vi "test_Set-Get Protocol ConvBox.vi"(8 "error in (no error)":errorcluster, 11 "TestCase in":refnum<class "Instrument Addon Scripting API Custom Device Unit Tests.lvclass">) -> (0 "error out":errorcluster, 3 "TestCase out":refnum<class "Instrument Addon Scripting API Custom Device Unit Tests.lvclass">)   [LabVIEW 2018, in "Instrument Addon Scripting API Custom Device Unit Tests.lvclass"]
uses:
  Instrument Addon Scripting API Custom Device Unit Tests.lvclass
  Addon/Support Libraries/Protocols.lvlibp/RS-xxx to GPIB ConvBox/RS-xxx to GPIB ConvBox.lvclass
  C:/Users/nitest/Git/NI VS Instrument Addon Fork/Source/Addon/Support Libraries/Protocols.lvlibp/Protocol Parent/Protocol Parent.lvclass
  Addon/Support Libraries/Protocols.lvlibp/TCP/TCP.lvclass
  Addon/Support Libraries/Protocols.lvlibp/RS-xxx to GPIB ConvBox/Data Access/Write Assert Ren with IFC.vi
  Addon/Support Libraries/Protocols.lvlibp/RS-xxx to GPIB ConvBox/Data Access/Write ConvBox Address.vi
  Addon/Support Libraries/Protocols.lvlibp/RS-xxx to GPIB ConvBox/Data Access/Write GPIB Address.vi
  Addon/Support Libraries/Protocols.lvlibp/RS-xxx to GPIB ConvBox/Data Access/Write IST bit sense.vi
  Addon/Support Libraries/Protocols.lvlibp/RS-xxx to GPIB ConvBox/Data Access/Write Port.vi
  Addon/Support Libraries/Protocols.lvlibp/RS-xxx to GPIB ConvBox/Data Access/Write System controller.vi
  Instrument Addon Scripting API Test Assets/Instrument Addon Scripting API Test Assets.lvclass
  <vilib>/addons/_JKI Toolkits/VI Tester/TestCase.llb/TestCase.lvclass
  APIs/Scripting API/Instrument Addon Scripting API.lvlib
  C:/Program Files (x86)/National Instruments/LabVIEW 2018/vi.lib/addons/_JKI Toolkits/VI Tester/TestCase.llb/TestCase.lvclass
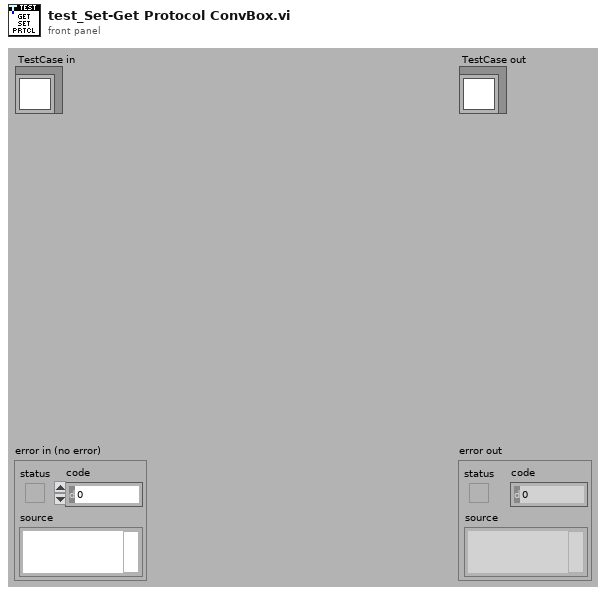
[diagram p1: front panel]
types:
  T1 = typedef "Custom Device API.lvlib/Custom Device Item Ref.ctl" = u64
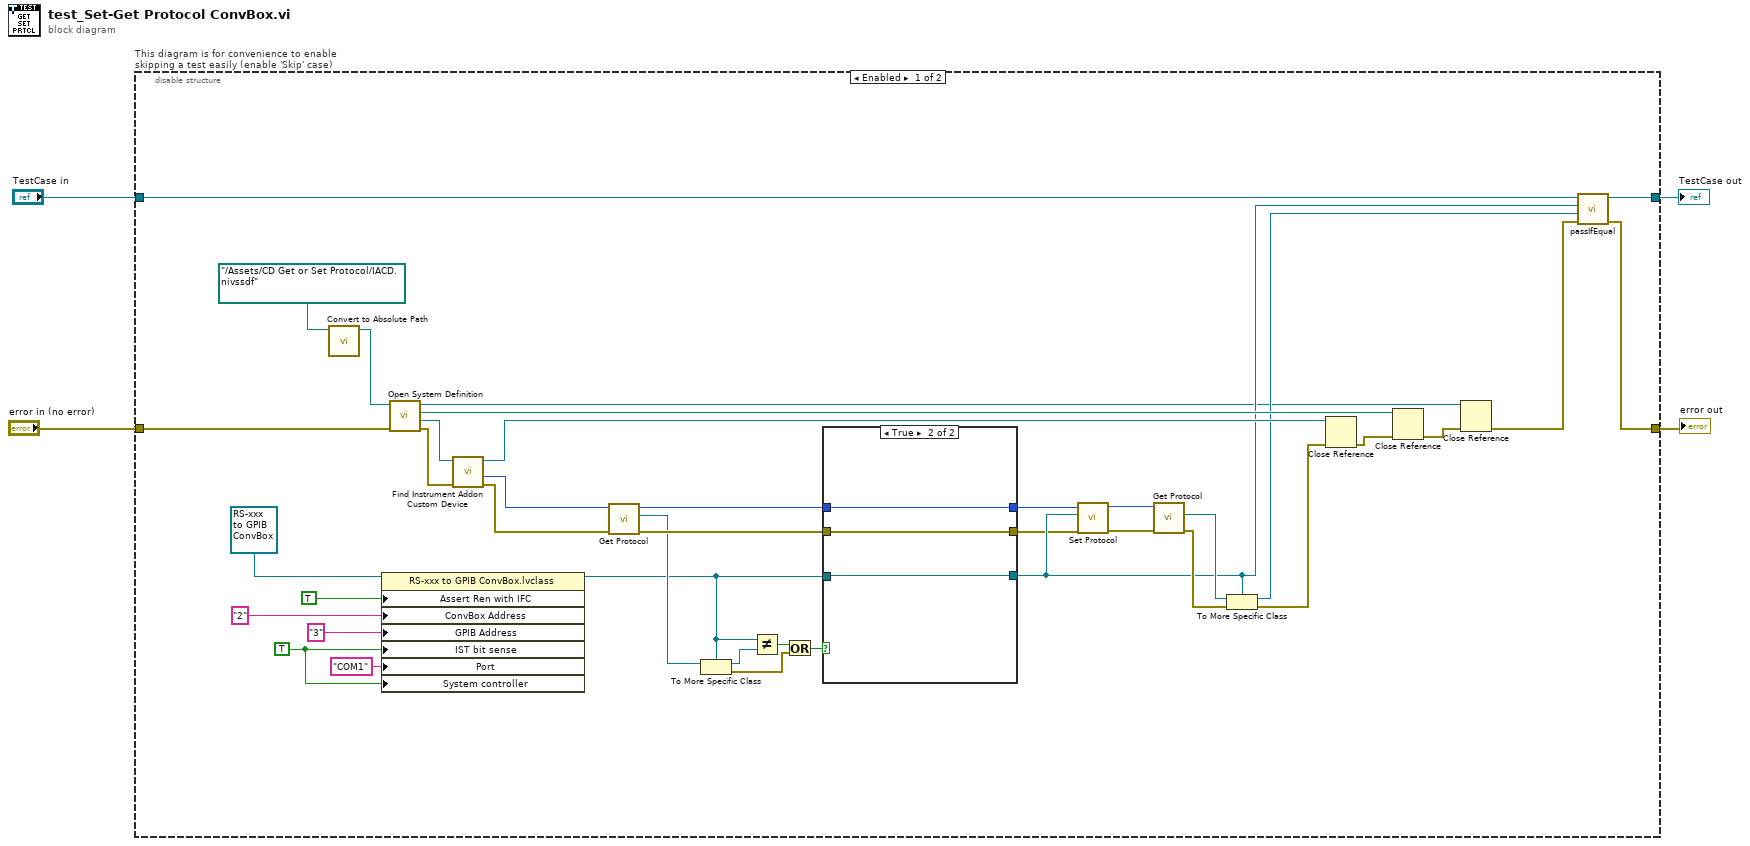
[diagram p0: block diagram]
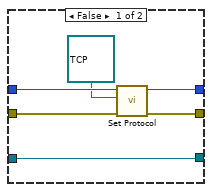
[diagram p2: hidden frame]
diagram:
  n1 = disable-structure "This diagram is for convenience to enable skipping a test easily (enable 'Skip' case)" shown="Enabled" {
    disable-tunnel: "TestCase in" -> [w30 w56]
    disable-tunnel: [w29 w54] -> w1
    disable-tunnel: [w26 w55] -> w3
    disable-tunnel: "error in (no error)" -> [w43 w53]
    frame Enabled {
      w20 = TRUE ("Assert Ren with IFC")
      n2 = call "Convert to Absolute Path.vi"("System Definition File"=path "../Assets/CD Get or Set Protocol/IACD.nivssdf" ("SDF file")) -> ("Absolute Path"=w41:path)  [unwired: 10 in]
      n3 = property class="RS-xxx to GPIB ConvBox.lvclass"(reference=refnum<class "RS-xxx to GPIB ConvBox.lvclass"> refnum ("Protocols.lvlibp:RS-xxx to GPIB ConvBox.lvclass"), "Assert Ren with IFC"=TRUE, "ConvBox Address"="2", "GPIB Address"="3" ("ConvBox Address"), "IST bit sense"=w20, "Port"="COM1", "System controller"=w20) -> (reference out=w10:refnum<class "RS-xxx to GPIB ConvBox.lvclass">)  [unwired: 1 in, 1 out]
      n4 = call "Open System Definition.vi"("error in (no error)"=w43, "System Definition File"=w41) -> ("error out"=w38:errorcluster, "Target Refnum"=w37:refnum<k24>, "Root Refnum"=w40:refnum<k24>, "System Definition Refnum"=w6:refnum<k24>)  [unwired: 6 in]
      n5 = call "Find Instrument Addon Custom Device.vi"("error in"=w38, "target in"=w37) -> ("error out"=w12:errorcluster, "NodeID"=w11:u64, "target out"=w36:refnum<k24>)  [unwired: 7 in]
      n6 = call "Get Protocol.vi"("Error In"=w12, "Instrument Addon Refnum In"=w11) -> ("Error Out"=w14:errorcluster, "Protocol"=w13:refnum<class "Protocol Parent.lvclass">, "Instrument Addon Refnum Out"=w15:T1)  [unwired: 7 in]
      n7 = To More Specific Class(target class=w10, reference=w13) -> (specific class reference=w19:refnum<class "RS-xxx to GPIB ConvBox.lvclass">, error out=w17:errorcluster)  [unwired: 1 in]
      n8 = Not Equal?(x=w10, y=w19) -> (x != y?=w18:bool)
      n9 = Or(x=w18, y=w17) -> (x .or. y?=w16:bool)
      n10 = case shown="True" w16 {
        tunnel: w15 -> [w47 w52]
        tunnel: w14 -> [w49 w51]
        tunnel: [w48 w51] -> w7
        tunnel: [w45 w52] -> w9
        tunnel: w10 -> [w44 w50]
        tunnel: [w44 w50] -> w8
        frame False {
          n11 = call "Set Protocol.vi"("Error In"=w49, "Protocol in"=refnum<class "TCP.lvclass"> refnum ("Protocols.lvlibp:TCP.lvclass"), "Instrument Addon Refnum In"=w47) -> ("Error Out"=w48:errorcluster, "Instrument Addon Refnum Out"=w45:T1)  [unwired: 7 in]
        }
        frame True {
        }
      }
      n12 = call "Set Protocol.vi"("Error In"=w7, "Protocol in"=w8, "Instrument Addon Refnum In"=w9) -> ("Error Out"=w34:errorcluster, "Instrument Addon Refnum Out"=w35:T1)  [unwired: 7 in]
      n13 = call "Get Protocol.vi"("Error In"=w34, "Instrument Addon Refnum In"=w35) -> ("Error Out"=w32:errorcluster, "Protocol"=w33:refnum<class "Protocol Parent.lvclass">)  [unwired: 7 in, 1 out]
      n14 = To More Specific Class(target class=w8, reference=w33, error in=w32) -> (specific class reference=w28:refnum<class "RS-xxx to GPIB ConvBox.lvclass">, error out=w31:errorcluster)
      n15 = Close Reference(reference=w36, error in (no error)=w31) -> (error out=w39:errorcluster)
      n16 = Close Reference(reference=w40, error in (no error)=w39) -> (error out=w5:errorcluster)
      n17 = Close Reference(reference=w6, error in (no error)=w5) -> (error out=w27:errorcluster)
      n18 = call-dynamic "passIfEqual.vi"("error in (no error)"=w27, "y"=w28, "x"=w8, "TestCase in"=w30) -> ("error out"=w26:errorcluster, "TestCase out"=w29:refnum<class "Instrument Addon Scripting API Custom Device Unit Tests.lvclass">)  [unwired: 6 in]
    }
    frame Disabled {
      # "skip test result while test is under development"
      n19 = call <vilib>:"skip.vi"("error in (no error)"=w53, "TestCase in"=w56) -> ("error out"=w55:errorcluster, "TestCase out"=w54:refnum<class "Instrument Addon Scripting API Custom Device Unit Tests.lvclass">)  [unwired: 8 in]
    }
  }
  "error out" <- w3
  "TestCase out" <- w1
